vi "gaussmeter_header.vi"() -> ()   [LabVIEW 2016]
panel:
  out "Gaussmeter Header":string
  out "error IO":errorcluster
  in  "Gaussmeter Number":u8
  in  "Probe Serial Number":string
  in  "Gaussmeter On/Off":bool
  in  "Probe Sensitivity":dbl
  in  "Probe Type":u16
  in  "error in (no error)":errorcluster
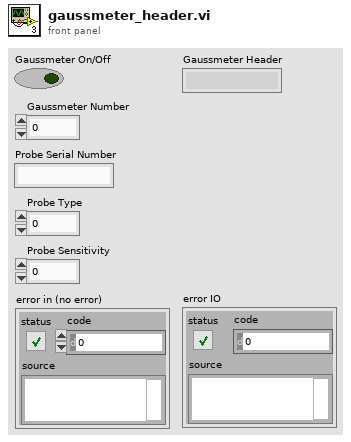
[diagram p1: front panel]
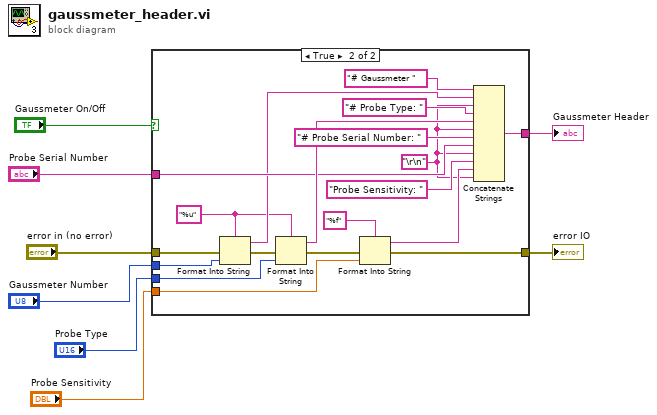
[diagram p0: block diagram]
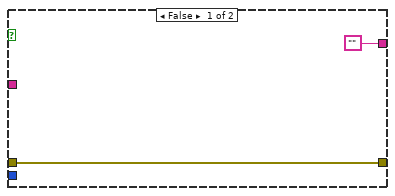
[diagram p2: hidden frame]
diagram:
  n1 = case shown="True" "Gaussmeter On/Off" {
    tunnel: "Probe Type" -> [_ w28]
    tunnel: ["" w29] -> w1
    tunnel: "Probe Sensitivity" -> [_ w27]
    tunnel: [w9 w26] -> w3
    tunnel: "error in (no error)" -> [w9 w16]
    tunnel: "Probe Serial Number" -> [_ w20]
    tunnel: "Gaussmeter Number" -> [_ w13]
    frame False {
    }
    frame True {
      w11 = "%u" ("format string")
      w18 = "\r\n"
      n2 = Format Into String(format string=w11, error in=w16, w13) -> (resulting string=w14:string, error out=w15:errorcluster)  [unwired: 1 in]
      n3 = Format Into String(format string=w11, error in=w15, w28) -> (resulting string=w21:string, error out=w25:errorcluster)  [unwired: 1 in]
      n4 = Format Into String(format string="%f", error in=w25, w27) -> (resulting string=w19:string, error out=w26:errorcluster)  [unwired: 1 in]
      n5 = Concatenate Strings("# Gaussmeter ", w14, w18, "# Probe Type: ", w21, w18, "# Probe Serial Number: ", w20, w18, "Probe Sensitivity: ", w19, w18) -> (w29:string)
    }
  }
  "error IO" <- w3
  "Gaussmeter Header" <- w1
